vi "Clear Radix Visible.vi"   [LabVIEW 2019]
doc: "VI for resetting the Radix Visible and Display Style Visible settings in the Test Target VI."
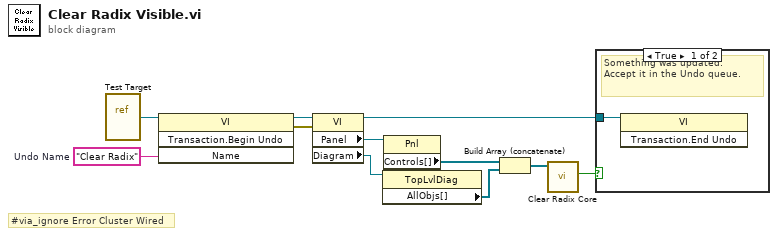
[diagram p0: block diagram]
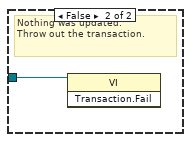
[diagram p2: hidden frame]
diagram:
  w6 = "Clear Radix"  # Undo Name
  # "#via_ignore Error Cluster Wired"
  n1 = vi-ref "Test Target.vi"() -> (w4:refnum<vi>)
  n2 = invoke on="Invoke Node" class="VI" method="Transaction.Begin Undo"(reference=w4, "Name"=w6) -> (reference out=w5:refnum<vi>, error out=w11:errorcluster)  [unwired: 2 in, 2 out]
  n3 = property on="Property Node" class="VI"(reference=w5, error in=w11) -> (reference out=w3:refnum<vi>, "Panel"=w10:refnum<vi>, "Diagram"=w9:refnum<vi>)  [unwired: 1 out]
  n4 = property on="Property Node" class="TopLvlDiag"(reference=w9) -> ("AllObjs[]"=w7:refnum<vi>[])  [unwired: 1 in, 2 out]
  n5 = property on="Property Node" class="Pnl"(reference=w10) -> ("Controls[]"=w8:refnum<vi>[])  [unwired: 1 in, 2 out]
  n6 = Build Array (concatenate)(w8, w7) -> (w2:refnum<vi>[])
  n7 = call "Clear Radix Core.vi"("GObjects"=w2) -> ("Successful"=w1:bool)  [unwired: 10 in]
  n8 = case shown="True" w1 {
    tunnel: w3 -> [w12 w13]
    frame True {
      # "Something was updated.\nAccept it in the Undo queue."
      n9 = invoke on="Invoke Node" class="VI" method="Transaction.End Undo"(reference=w12) -> ()  [unwired: 2 in, 3 out]
    }
    frame False {
      # "Nothing was updated.\nThrow out the transaction."
      n10 = invoke on="Invoke Node" class="VI" method="Transaction.Fail"(reference=w13) -> ()  [unwired: 2 in, 3 out]
    }
  }
